vi "CreateXL_Workbook.vi"(8 "error in":errorcluster, 10 "path":path, 11 "Refnum Cluster In":T1) -> (0 "error out":errorcluster, 3 "Refnum Cluster Out":T2)   [LabVIEW 2017, in "excel_configuration.lvlib"]
uses:
  excel_configuration.lvlib
  f7b3d193-71f7-44bb-8cd8-d9715c05a7d6.vi
  <vilib>/Utility/error.llb/Clear Errors.vi
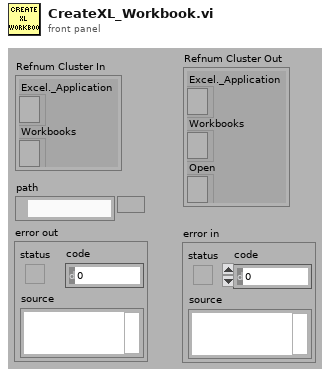
[diagram p1: front panel]
types:
  T1 = cluster{"Excel._Application":refnum<k7>, "Workbooks":refnum<k7>}
  T2 = cluster{"Excel._Application":refnum<k7>, "Workbooks":refnum<k7>, "Open":refnum<k7>}
  T3 = enum32{"existing file", "new file", "new or existing file", "existing dir", "new dir", "new or existing dir", "existing file (use LLBs)", "new file (use LLBs)", "new or existing file (use LLBs)", "new or existing file or directory (use LLBs)"}
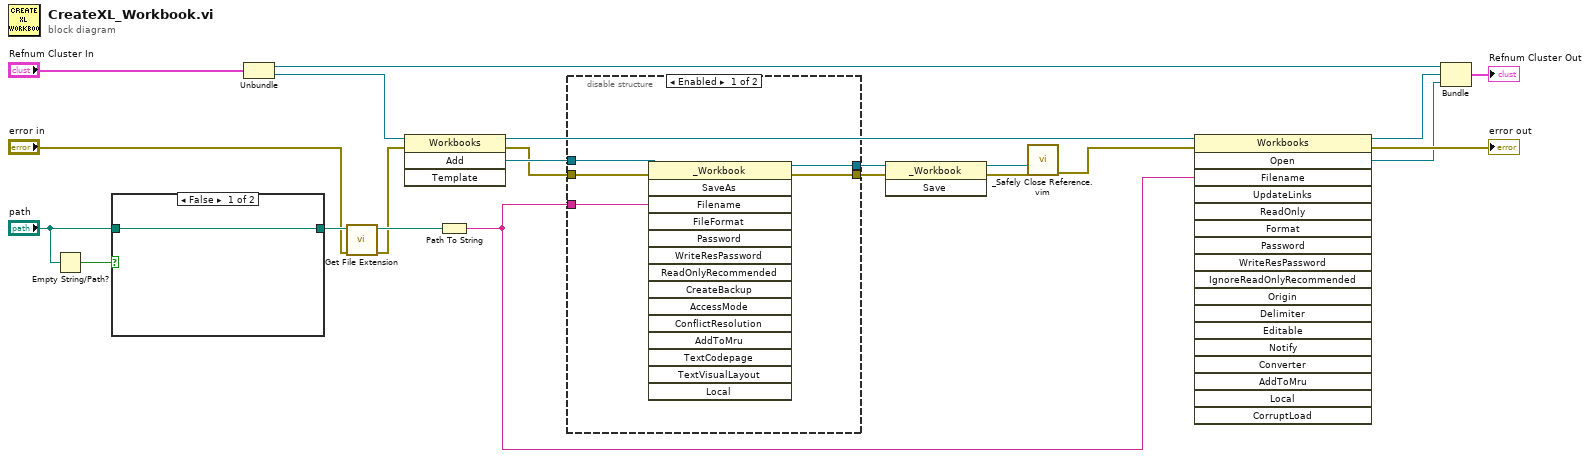
[diagram p0: block diagram]
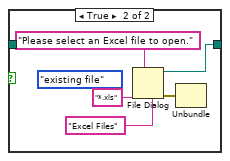
[diagram p3: hidden frame]
diagram:
  n1 = Empty String/Path?(string/path="path") -> (empty?=w19:bool)
  n2 = case shown="False" w19 {
    tunnel: "path" -> [w23 _]
    tunnel: [w23 w28] -> w8
    frame False {
    }
    frame True {
      (unwired) T3."existing file" ("select mode (2)")
      n3 = File Dialog(4:"Excel Files" ("pattern label"), 6:"*.xls" ("pattern"), 7:"Please select an Excel file to open." ("prompt")) -> (0:w24:errorcluster, 3:w28:path)  [unwired: 4 in, 2 out]
      n4 = Unbundle(w24) -> ()  [unwired: 3 out]
    }
  }
  n5 = Unbundle("Refnum Cluster In") -> ("Excel._Application"=w22:refnum<k7>, "Workbooks"=w20:refnum<k7>)
  n6 = call <vilib>:"Get File Extension.vi"("error in (no error)"="error in", "file"=w8) -> ("error out"=w5:errorcluster, "dup file"=w7:path)  [unwired: 5 in, 3 out]
  n7 = invoke class="Workbooks" method="Add"(reference=w20, error in=w5) -> (reference out=w15:refnum<k7>, error out=w16:errorcluster, "Add"=w17:refnum<k7>)  [unwired: 2 in, 1 out]
  n8 = Path To String(path=w7) -> (string=w9:string)
  n9 = disable-structure shown="Enabled" {
    disable-tunnel: w17 -> [w30 w35]
    disable-tunnel: w16 -> [w33 w34]
    disable-tunnel: w9 -> [w29 _]
    disable-tunnel: [w32 w34] -> w4
    disable-tunnel: [w31 w35] -> w3
    frame Enabled {
      n10 = invoke class="_Workbook" method="SaveAs"(reference=w30, error in=w33, "Filename"=w29) -> (reference out=w31:refnum<k7>, error out=w32:errorcluster)  [unwired: 12 in, 13 out]
    }
    frame Disabled {
    }
  }
  n11 = invoke class="_Workbook" method="Save"(reference=w3, error in=w4) -> (reference out=w1:refnum<k7>, error out=w2:errorcluster)  [unwired: 1 in, 1 out]
  n12 = call "_Safely Close Reference.vim"("error in (no error)"=w2, "Automation Refnum in"=w1) -> ("error out"=w13:errorcluster)  [unwired: 9 in]
  n13 = invoke class="Workbooks" method="Open"(reference=w15, error in=w13, "Filename"=w9) -> (reference out=w14:refnum<k7>, error out=→"error out":errorcluster, "Open"=w11:refnum<k7>)  [unwired: 15 in, 15 out]
  n14 = Bundle("Excel._Application"=w22, "Workbooks"=w14, "Open"=w11) -> (→"Refnum Cluster Out":T2)  [unwired: 1 in]
